vi "filter.ip.vi"(9 "reset":bool, 10 "debug":bool) -> ()   [LabVIEW 2020]
uses:
  <vilib>/Platform/TimedLoop/XDataNode/XDataNode.xnode
  <vilib>/Platform/TimedLoop/XDataNode/nitl_modes.ctl
  <vilib>/Platform/TimedLoop/XDataNode/XDNodeRunTimeDep.lvlib
  <vilib>/Platform/TimedLoop/XDataNode/wakeup.ctl
  <vilib>/Platform/TimedLoop/XDataNode/timing_clust.ctl
  <vilib>/rvi/LocalResourceManager/LocalResourceManager.xnode
  <vilib>/rvi/DataTransferAndStorage/Container/XNode/niFpgaContainer.xnode
  <vilib>/rvi/FIFO/Fifo_Resource/niFpgaFifoEmulationRefIn.vi
  <vilib>/rvi/FIFO/Fifo_Resource/nirvififoEmulationRead.vi
  ticker.slot.ctl
  Market.Data.Common/fpga/orderbook.command.ctl
  Market.Data.Common/fpga/fpganow.common.fpga.lvlib
  Market.Data.Common/fpga/orderbook.command.type.ctl
  <vilib>/rvi/DataTransferAndStorage/Container/Common/niFpgaContainerGetUniqueNameForEmu.vi
  <vilib>/rvi/DataTransferAndStorage/Container/Common/niFpgaContainerSetEmuInfo.vi
  <vilib>/rvi/eio/common/nirviEmuReportErrorAndStop.vi
  <vilib>/rvi/FIFO/Fifo_Resource/nirvififoEmulationWrite.vi
panel:
  out "Debug.Data":T1
  in  "Command.In.Remove":bool
  in  "Command.In.Edit":bool
  in  "Command.In.Add":bool
  in  "Command.In.Seq.No":u32
  out "Command.Out.Seq.No":u32
  in  "Command.In.nanoseconds":u64
  in  "Command.In.seconds":u64
  in  "Command.In.remaining.qty":u32
  in  "Command.In.canceled.qty":u32
  in  "Command.In.executed.qty":u32
  in  "Command.In.price":u64
  in  "Command.In.symbol":u64
  in  "Command.In.quantity":u32
  in  "Command.In.orderId":u64
  in  "Command.In.side":u8
  in  "Command.In.type":T2
  out "Command.Out.Remove":bool
  out "Command.Out.Edit":bool
  out "Command.Out.Add":bool
  out "Command.Out.nanoseconds":u64
  out "Command.Out.seconds":u64
  out "Command.Out.remaining.qty":u32
  out "Command.Out.canceled.qty":u32
  out "Command.Out.executed.qty":u32
  out "Command.Out.price":u64
  out "Command.Out.symbol":u64
  out "Command.Out.quantity":u32
  out "Command.Out.orderId":u64
  out "Command.Out.side":u8
  out "Command.Out.type":T3(ring)
  in  "Command.In.Valid":bool
  out "State.Out.Valid":bool
  out "State.Out.Quantity":u64
  out "State.Out.OrderId":u64
  out "Command.Out.Valid":bool
  out "Debug.Valid":bool
  in  "Symbol.Valid":bool
  in  "Symbol":u64
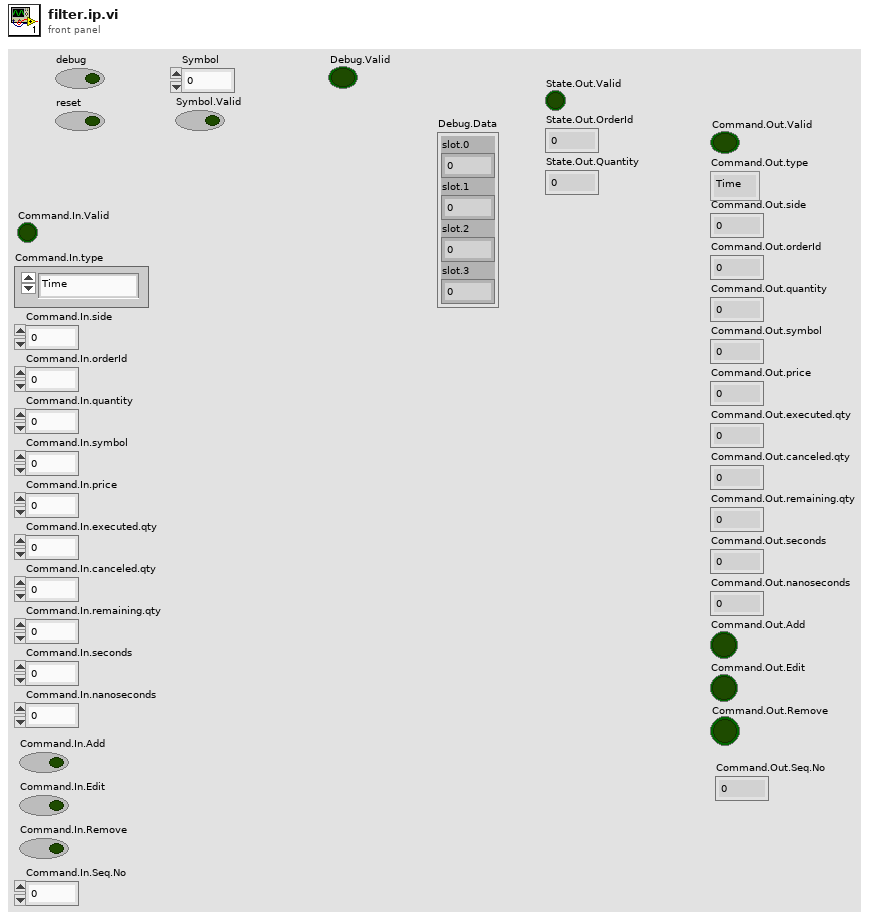
[diagram p1: front panel]
types:
  T1 = cluster{"slot.0":u64, "slot.1":u64, "slot.2":u64, "slot.3":u64}
  T2 = typedef "fpganow.common.fpga.lvlib/orderbook.command.type.ctl" = enum8{"Time", "AddOrder", "OrderExecuted", "OrderExecutedAtPrice", "ReduceSize", "ModifyOrder", "DeleteOrder", "Get.Everything", "Get.All.Orders", "Get.Top"}
  T3 = enum8{"Time", "AddOrder", "OrderExecuted", "OrderExecutedAtPrice", "ReduceSize", "ModifyOrder", "DeleteOrder", "Get.Everything", "Get.All.Orders", "Get.Top"}
  T4 = typedef "XDNodeRunTimeDep.lvlib/timing_clust.ctl" = cluster{"Expected End [f-1]":u64, "Actual End [f-1]":u64, "Finished Late? [f-1]":bool, "Expected End [i-1]":u64, "Actual End [i-1]":u64, "Finished Late? [i-1]":bool, "Expected Start [i]":u64, "Actual Start [i]":u64, "Expected Start [f]":u64, "Actual Start [f]":u64, "Source Name":string, "Structure Name":string, "Period":i64, "Deadline":i64, "Offset":i64, "Start":i64, "Priority":i32, "Timeout":i32, "Mode":T5, "Wakeup Reason":T6, "Error":errorcluster, "Source Type":string, "Secondary Source Type":string, "Global End Time":u64, "Global Start Time":u64, "Frame Duration":u64, "Iteration Duration":u64, "Assigned CPU":i32, "I/O Scan Engine Mode":u32}
  T5 = typedef "XDNodeRunTimeDep.lvlib/nitl_modes.ctl" = enum32{"No Change", "Process missed periods, maintain original phase", "Discard missed periods, maintain original phase", "Process missed periods, ignore original phase", "Discard missed periods, ignore original phase"}
  T6 = typedef "XDNodeRunTimeDep.lvlib/wakeup.ctl" = enum32{"Normal", "Aborted", "Asynchronous wakeup", "Timing source error", "Timed loop error", "Timeout"}
  T7 = typedef "fpganow.common.fpga.lvlib/orderbook.command.ctl" = cluster{"type":T2, "side":u8, "orderId ":u64, "quantity":u32, "symbol":u64, "price":u64, "executed.qty":u32, "canceled.qty":u32, "remaining.qty":u32, "seconds":u64, "nanoseconds":u64, "Add":bool, "Edit":bool, "Remove":bool, "seq no":u32, "recv.time":u64, "parse.time":u64}
  T8 = typedef "ticker.slot.ctl" = cluster{"Symbol":u64}
  T9 = cluster{"type":enum8{"Time", "AddOrder", "OrderExecuted", "OrderExecutedAtPrice", "ReduceSize", "ModifyOrder", "DeleteOrder", "Get.Everything", "Get.All.Orders", "Get.Top"}, "side":u8, "orderId ":u64, "quantity":u32, "symbol":u64, "price":u64, "executed.qty":u32, "canceled.qty":u32, "remaining.qty":u32, "seconds":u64, "nanoseconds":u64, "Add":bool, "Edit":bool, "Remove":bool, "seq no":u32}
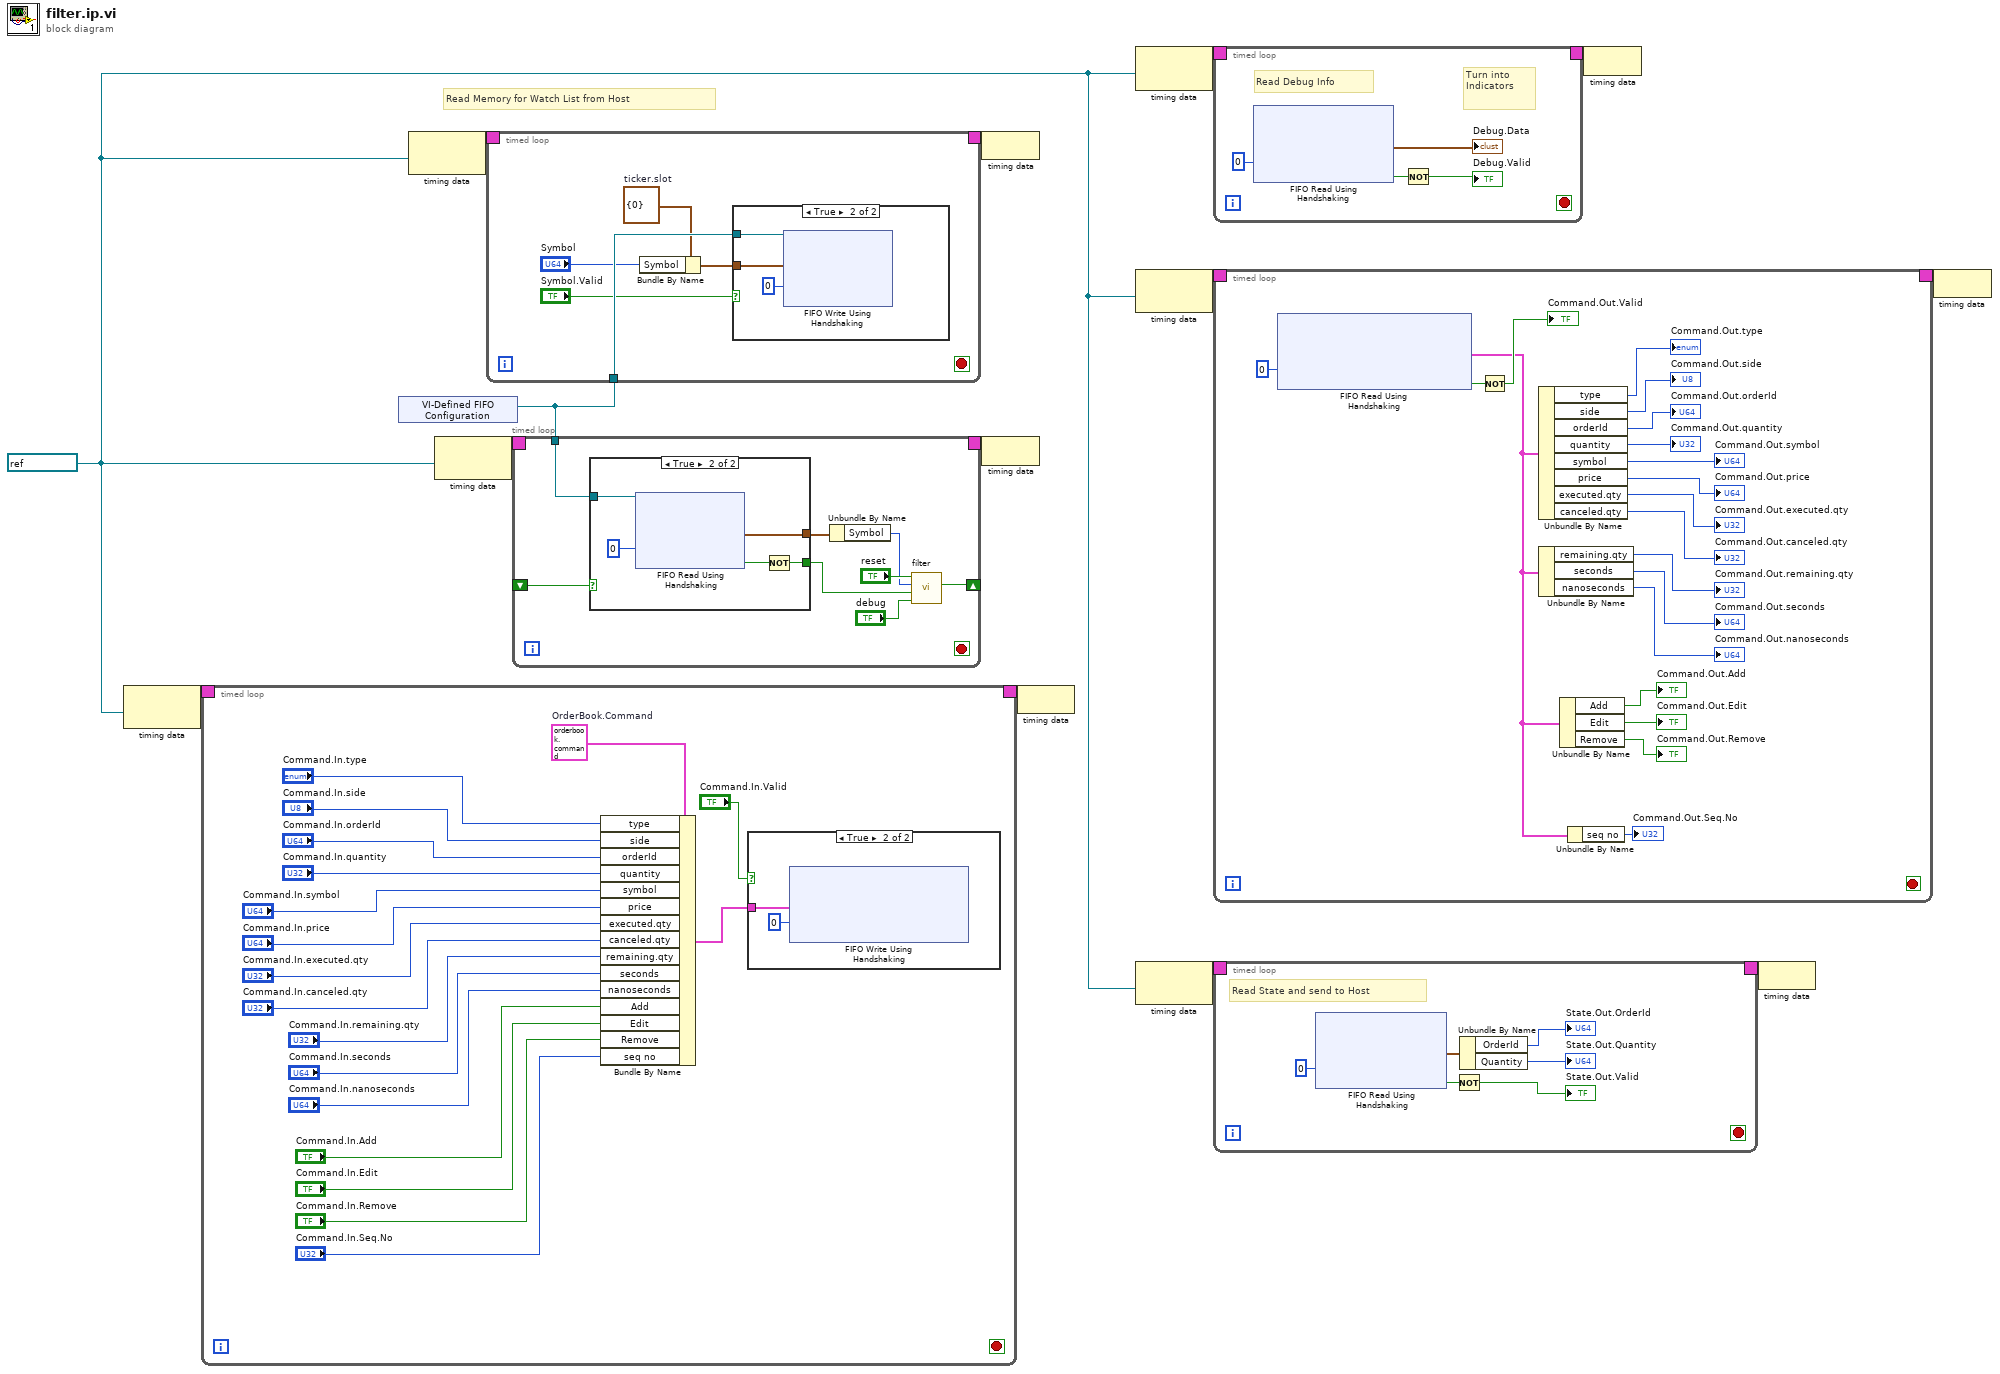
[diagram p0: block diagram]
diagram:
  w1 = refnum<k21> "100MHz" ("Source Name")
  # "Read Memory for Watch List from Host"
  n1 = node-c288(w1) -> (w7:T4)
  n2 = timed-loop {
    timing: w7 -> [_]
    timing-out: [_] -> w6
    stop <- _ stop-if-true
    w32 = T7 {"type"=enum."AddOrder", "side"=0, "orderId "=0, "quantity"=0, "symbol"=0, "price"=0, "executed.qty"=0, "canceled.qty"=0, "remaining.qty"=0, "seconds"=0, "nanoseconds"=0, "Add"=FALSE, "Edit"=FALSE, "Remove"=FALSE, "seq no"=0, "recv.time"=0, "parse.time"=0}  # OrderBook.Command
    n3 = Bundle By Name(cluster=w32, "type"="Command.In.type", "side"="Command.In.side", "orderId"="Command.In.orderId", "quantity"="Command.In.quantity", "symbol"="Command.In.symbol", "price"="Command.In.price", "executed.qty"="Command.In.executed.qty", "canceled.qty"="Command.In.canceled.qty", "remaining.qty"="Command.In.remaining.qty", "seconds"="Command.In.seconds", "nanoseconds"="Command.In.nanoseconds", "Add"="Command.In.Add", "Edit"="Command.In.Edit", "Remove"="Command.In.Remove", "seq no"="Command.In.Seq.No") -> (w31:T7)
    n4 = case shown="True" "Command.In.Valid" {
      tunnel: w31 -> [_ w34]
      frame False {
      }
      frame True {
        n5 = xnode ("FIFO Write Using Handshaking")("Element"=w34, "Timeout"=0) -> ()  [unwired: 1 in, 2 out]
      }
    }
  }
  n6 = xnode "VI-Defined FIFO Configuration"() -> ("FIFO Out"=w10:refnum<k21>)
  n7 = node-c288(w1) -> (w12:T4)
  n8 = node-c288(w1) -> (w14:T4)
  n9 = timed-loop {
    timing: w12 -> [_]
    timing-out: [_] -> w11
    tunnel: w10 -> [w41]
    stop <- _ stop-if-true
    w40 = T8 {"Symbol"=0}  # ticker.slot
    n10 = Bundle By Name(cluster=w40, "Symbol"="Symbol") -> (w39:T8)
    n11 = case shown="True" "Symbol.Valid" {
      tunnel: w41 -> [_ w44]
      tunnel: w39 -> [_ w43]
      frame False {
      }
      frame True {
        n12 = xnode ("FIFO Write Using Handshaking")("Element"=w43, "Timeout"=0, "FIFO In"=w44) -> ()  [unwired: 2 out]
      }
    }
  }
  n13 = timed-loop {
    timing: w14 -> [_]
    timing-out: [_] -> w13
    tunnel: w10 -> [w54]
    shift-right: [w49] -> _
    shift-left: _ -> [w47]
    stop <- _ stop-if-true
    n14 = case shown="True" w47 {
      tunnel: w54 -> [_ w59]
      tunnel: [_ w58] -> w53
      tunnel: [_ w55] -> w51
      frame False {
      }
      frame True {
        n15 = xnode ("FIFO Read Using Handshaking")("Timeout"=0, "FIFO In"=w59) -> ("Element"=w58:cluster{"Symbol":u64}, "Timed Out?"=w56:bool)  [unwired: 1 out]
        n16 = Not(x=w56) -> (.not. x?=w55:bool)
      }
    }
    n17 = Unbundle By Name(w53) -> ("Symbol"=w48:u64)
    n18 = call "filter.vi"("debug"="debug", "conf.valid"=w51, "conf"=w48, "reset"="reset") -> ("Ready.for.Configuration.Input"=w49:bool)  [unwired: 6 in, 1 out]
  }
  n19 = node-c288(w11) -> ()
  n20 = node-c288(w13) -> ()
  n21 = node-c288(w6) -> ()
  n22 = node-c288(w1) -> (w9:T4)
  n23 = node-c288(w1) -> (w5:T4)
  n24 = node-c288(w1) -> (w3:T4)
  n25 = timed-loop {
    timing: w9 -> [_]
    timing-out: [_] -> w8
    stop <- _ stop-if-true
    # "Turn into \nIndicators"
    # "Read Debug Info"
    n26 = xnode ("FIFO Read Using Handshaking")("Timeout"=0) -> ("Element"=→"Debug.Data":T1, "Timed Out?"=w64:bool)  [unwired: 1 in, 1 out]
    n27 = Not(x=w64) -> (.not. x?=→"Debug.Valid":bool)
  }
  n28 = timed-loop {
    timing: w5 -> [_]
    timing-out: [_] -> w4
    stop <- _ stop-if-true
    n29 = xnode ("FIFO Read Using Handshaking")("Timeout"=0) -> ("Element"=w69:T9, "Timed Out?"=w85:bool)  [unwired: 1 in, 1 out]
    n30 = Not(x=w85) -> (.not. x?=→"Command.Out.Valid":bool)
    n31 = Unbundle By Name(w69) -> ("type"=→"Command.Out.type":T3, "side"=→"Command.Out.side":u8, "orderId"=→"Command.Out.orderId":u64, "quantity"=→"Command.Out.quantity":u32, "symbol"=→"Command.Out.symbol":u64, "price"=→"Command.Out.price":u64, "executed.qty"=→"Command.Out.executed.qty":u32, "canceled.qty"=→"Command.Out.canceled.qty":u32)
    n32 = Unbundle By Name(w69) -> ("remaining.qty"=→"Command.Out.remaining.qty":u32, "seconds"=→"Command.Out.seconds":u64, "nanoseconds"=→"Command.Out.nanoseconds":u64)
    n33 = Unbundle By Name(w69) -> ("Add"=→"Command.Out.Add":bool, "Edit"=→"Command.Out.Edit":bool, "Remove"=→"Command.Out.Remove":bool)
    n34 = Unbundle By Name(w69) -> ("seq no"=→"Command.Out.Seq.No":u32)
  }
  n35 = timed-loop {
    timing: w3 -> [_]
    timing-out: [_] -> w2
    stop <- _ stop-if-true
    # "Read State and send to Host"
    n36 = xnode ("FIFO Read Using Handshaking")("Timeout"=0) -> ("Element"=w94:cluster{"OrderId":u64, "Quantity":u64}, "Timed Out?"=w92:bool)  [unwired: 1 in, 1 out]
    n37 = Not(x=w92) -> (.not. x?=→"State.Out.Valid":bool)
    n38 = Unbundle By Name(w94) -> ("OrderId"=→"State.Out.OrderId":u64, "Quantity"=→"State.Out.Quantity":u64)
  }
  n39 = node-c288(w8) -> ()
  n40 = node-c288(w2) -> ()
  n41 = node-c288(w4) -> ()
